vi "setPmwOut.vi"(0 "SEDSpectrometer in":refnum<class "SEDSpectrometer.lvclass">, 5 "Device":i32, 7 "PortId":u8, 9 "Freq":u32, 11 "error in (no error)":errorcluster, 12 "Duty":u8) -> (4 "SEDSpectrometer out":refnum<class "SEDSpectrometer.lvclass">, 6 "Output Value":i32, 15 "error out":errorcluster)   [LabVIEW 2016, in "SEDSpectrometer.lvclass"]
uses:
  SEDSpectrometer.lvclass
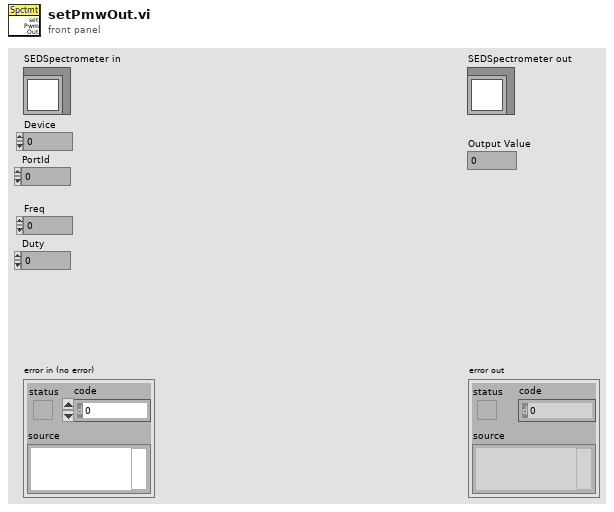
[diagram p1: front panel]
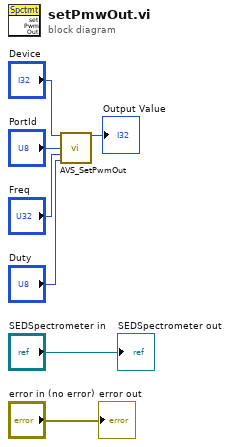
[diagram p0: block diagram]
diagram:
  n1 = call "AVS_SetPwmOut.vi"("a_hDevice"="Device", "a_PortId"="PortId", "a_Freq"="Freq", "a_Duty"="Duty") -> ("Output Value"=→"Output Value":i32)  [unwired: 11 in]
  "error out" <- "error in (no error)"
  "SEDSpectrometer out" <- "SEDSpectrometer in"
